vi "Write Double.vi"(8 "error in (no error)":errorcluster, 10 "Double":dbl, 11 "Event in":refnum<class "Event Double.lvclass">) -> (0 "error out":errorcluster, 3 "Event out":refnum<class "Event Double.lvclass">)   [LabVIEW 2023, in "MVC Actors.lvlib" / "Event Double.lvclass"]
uses:
  Event Double.lvclass
  Event Double.lvclass/Event Double.ctl
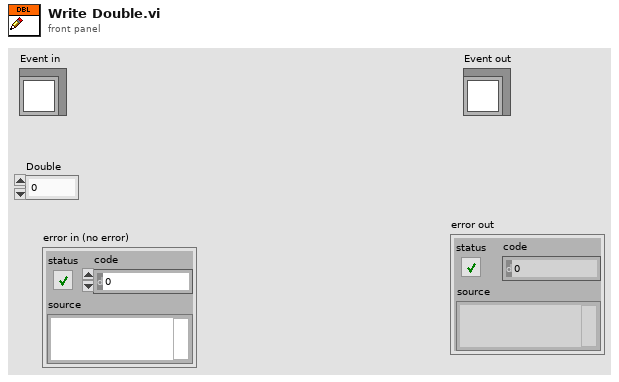
[diagram p1: front panel]
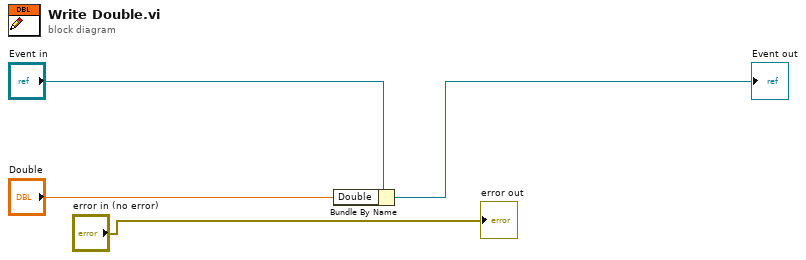
[diagram p0: block diagram]
diagram:
  n1 = Bundle By Name(cluster="Event in", "Double"="Double") -> (→"Event out":refnum<class "Event Double.lvclass">)
  "error out" <- "error in (no error)"
